vi "Write TestResultInformation.vi"(8 "error in (no error)":errorcluster, 10 "TestResultInformation":T1, 11 "TestResultInformation in":refnum<class "TestResultInformation.lvclass">) -> (0 "error out":errorcluster, 3 "TestResultInformation out":refnum<class "TestResultInformation.lvclass">)   [LabVIEW 2019, in "TestEngine.lvlib" / "TestResultInformation.lvclass"]
uses:
  TestResultInformation.lvclass
  TestResultInformation.lvclass/TestResultInformation.ctl
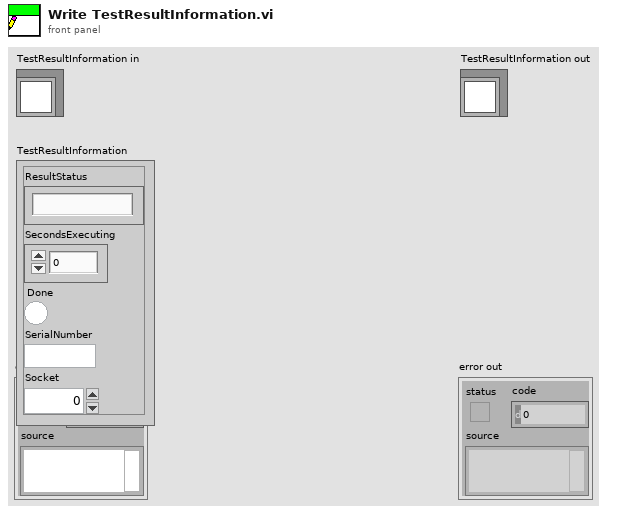
[diagram p1: front panel]
types:
  T1 = cluster{"ResultStatus":string, "SecondsExecuting":dbl, "Done":bool, "SerialNumber":string, "Socket":i32}
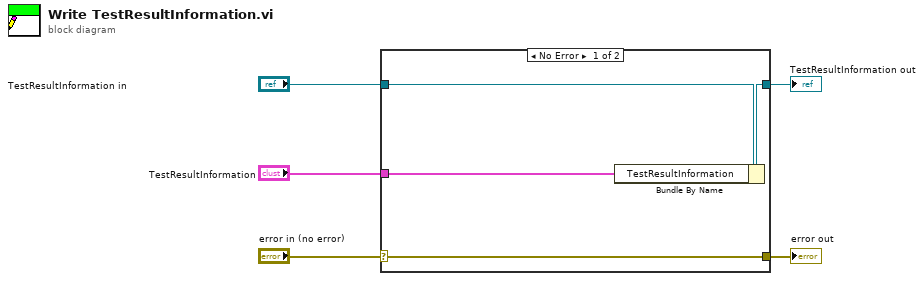
[diagram p0: block diagram]
diagram:
  n1 = case shown="No Error" "error in (no error)" {
    selector: "error in (no error)" -> [w9 w10]
    tunnel: [w9 w10] -> w4
    tunnel: [w7 w11] -> w2
    tunnel: "TestResultInformation in" -> [w8 w11]
    tunnel: "TestResultInformation" -> [w6 _]
    frame No Error {
      n2 = Bundle By Name(cluster=w8, "TestResultInformation"=w6) -> (w7:refnum<class "TestResultInformation.lvclass">)
    }
    frame Error {
    }
  }
  "error out" <- w4
  "TestResultInformation out" <- w2
